vi "testvi.vi"() -> ()   [LabVIEW 2011]
panel:
  in  "Numeric":dbl
  out "x+1":dbl
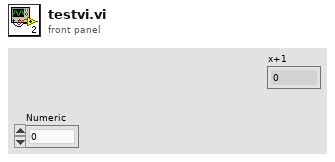
[diagram p1: front panel]
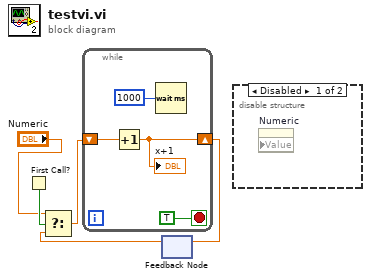
[diagram p0: block diagram]
diagram:
  n1 = First Call?() -> (First Call?: T/F=w5:bool)
  n2 = feedback #1() -> (w1:dbl)  [unwired: 1 in]
  n3 = Select(t="Numeric", s=w5, f=w1) -> (s? t:f=w3:dbl)
  n4 = while {
    shift-right: [w8] -> w2
    shift-left: w3 -> [w6]
    stop <- TRUE stop-if-true
    n5 = Increment(x=w6) -> (x+1=w8:dbl)
    "x+1" <- w8
    n6 = Wait (ms)(milliseconds to wait=u32 1000) -> ()  [unwired: 1 out]
  }
  n7 = feedback-in #1(w2) -> ()
  n8 = disable-structure shown="Disabled" {
    frame Disabled {
      n9 = property on="Numeric" class="DigNum (strict)" props=["Value"]() -> ()  [unwired: 3 in, 2 out]
    }
    frame Enabled {
    }
  }
